vi "rx_top.vi"(0 "Received IQ\nwaveform":cluster{"t0":dbl, "dt":dbl, "Y":cdb[]} {"Y" format="%.2g"; "dt" format="%.2g"; "t0" format="%.2g"}, 2 "Modulation Parameters":T4 {"RX Parameters"."RX Sample Rate" items=["4M"]}, 4 "# of Receive Iterations":u16=1, 6 "stop":bool, 7 "error in":errorcluster) -> (9 "Received IQ Graph":cluster{dbl[], dbl[]}(graph) caption="IQ Graph", 10 "Received Magnitude":dbl[](graph), 11 "Received Constellation Graph":T7(graph) caption="Constellation Graph", 12 "Received Phase":dbl[](graph), 13 "Received Eye Diagram":cluster{"t0":dbl, "dt":dbl, "Y":dbl[]}[](graph) caption="Eye Diagram", 14 "coerced carrier frequency (Hz)":dbl format="%#_6p", 15 "Received I":waveform(dbl)(graph), 16 "coerced bandwidth":dbl, 17 "Received Q":waveform(dbl)(graph), 18 "coerced gain (dB)":dbl format="%#_6f", 19 "Received Power Spectrum Density":dbl[](graph), 20 "Measured channel impairements":T2, 21 "symbol rate":dbl format="%#_6p", 22 "offset":i32, 23 "overhead offset":i32, 24 "bit-error rate":dbl, 25 "average \nbit-error rate":dbl, 26 "key bit sequence":u8[](array[numeric]), 27 "error out":errorcluster)   [LabVIEW 2012]
uses:
  EE 497/LABS/SDR/control_type_defs.llb/rx_hw params.ctl
  EE 497/LABS/SDR/control_type_defs.llb/Queues.ctl
  <vilib>/Analysis/baseanly.llb/Mean (DBL).vi
  gds_hw_config.lvlib
  <vilib>/addons/Modulation/niAMT.lvlib
  <vilib>/Analysis/NI_AALBase.lvlib
panel:
  in  "Queues":T1
  out "Packet Detected":bool
  in  "Configurations":T3(tab)
  in  "HW parameters":T5={"Device IP Address"="192.168.11.6", "Active Antenna"="RX1", "Carrier Frequency (Hz)"=915000000.0, "Gain (dB)"=10.0, "Trigger Level"=0.01, "Bandwidth (Hz)"=40000000.0, "Reference Position (%)"=10.0, "Capture Time (s)"=0.0004, "Simulate"=FALSE} {"Capture Time (s)" format="%.2p"; "Bandwidth (Hz)" format="%.2p"; "Trigger Level" format="%#.3p"; "Gain (dB)" format="%.2f"; "Carrier Frequency (Hz)" format="%.2p"}
  in  "RX Graphs":T6(tab)
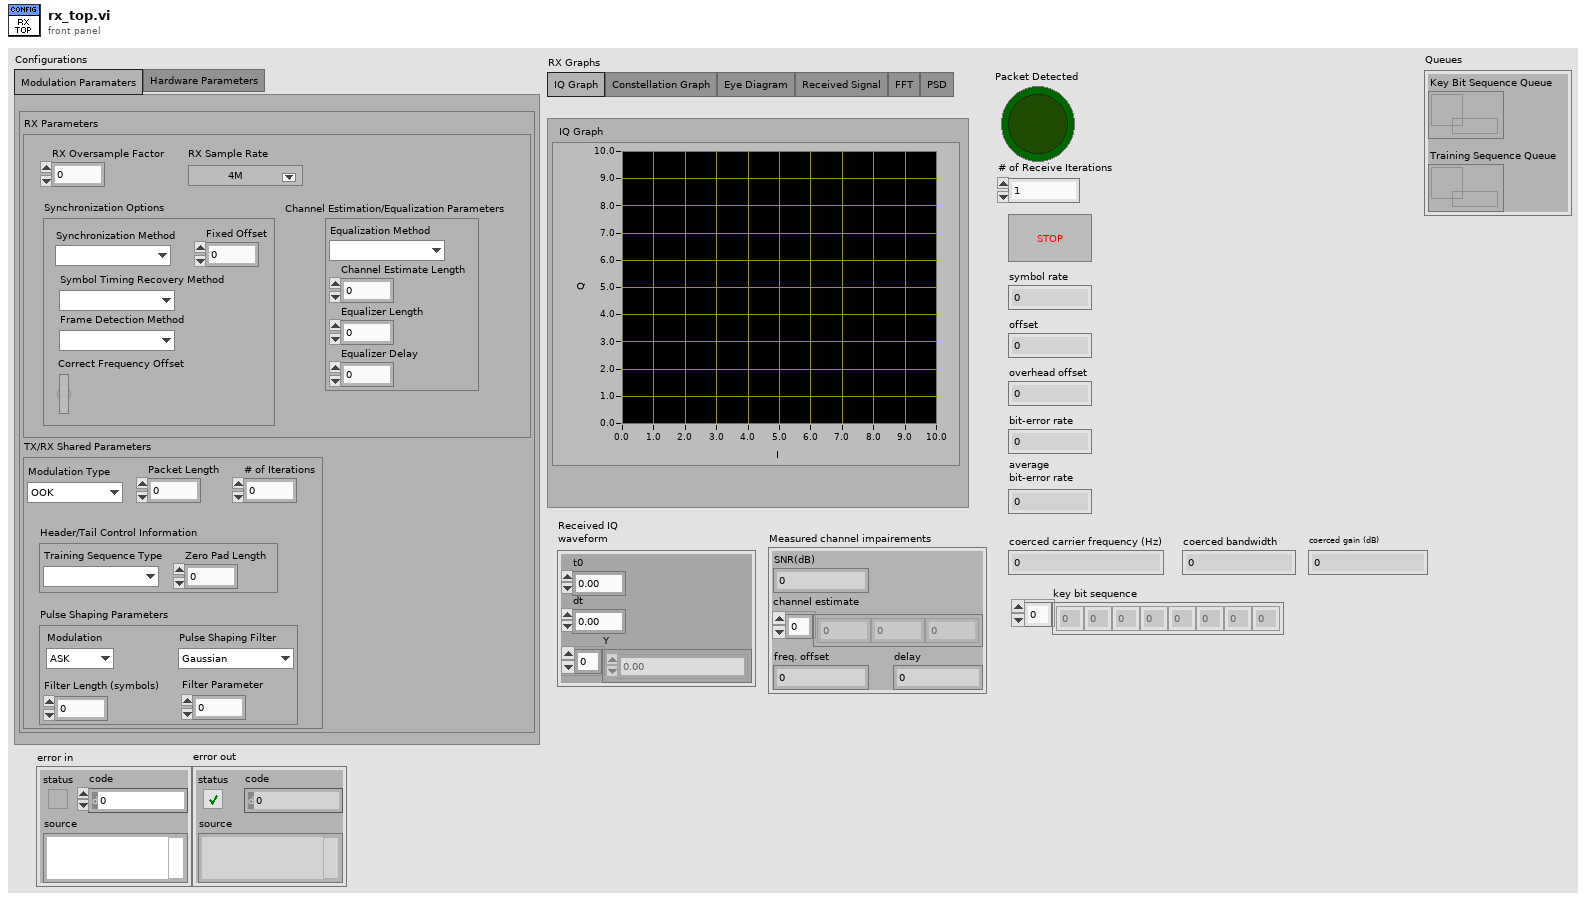
[diagram p1: front panel]
types:
  T1 = typedef "Queues.ctl" = cluster{"Key Bit Sequence Queue":refnum<queue>, "Training Sequence Queue":refnum<queue>}
  T2 = cluster{"SNR(dB)":dbl, "channel estimate":cdb[], "freq. offset":dbl, "delay":dbl}
  T3 = enum32{"Modulation Paramaters", "Hardware Parameters"}
  T4 = cluster{"RX Parameters":cluster{"RX Oversample Factor":dbl, "RX Sample Rate":dbl, "Synchronization Options":cluster{"Synchronization Method":enum16{""}, "Symbol Timing Recovery Method ":enum16{""}, "Fixed Offset":dbl, "Frame Detection Method":enum16{""}, "Correct Frequency Offset":bool}, "Channel Estimation/Equalization Parameters":cluster{"Equalization Method":enum16{""}, "Channel Estimate Length":dbl, "Equalizer Length":dbl, "Equalizer Delay":dbl}}, "TX/RX Shared Parameters":cluster{"Modulation Type":enum16{"OOK", "FSK"}, "Packet Length":dbl, "# of Iterations":dbl, "Pulse Shaping Parameters":cluster{"Modulation":enum16{"ASK", "FSK", "PSK", "QAM", "MSK", "PAM"}, "Pulse Shaping Filter":enum16{"Gaussian"}, "Filter Length (symbols)":dbl, "Filter Parameter":dbl}, "Header/Tail Control Information":cluster{"Training Sequence Type":enum16{""}, "Zero Pad Length":dbl}}}
  T5 = typedef "rx_hw params.ctl" = cluster{"Device IP Address":refnum<k15>, "Active Antenna":string, "Carrier Frequency (Hz)":dbl, "Gain (dB)":dbl, "Trigger Level":dbl, "Bandwidth (Hz)":dbl, "Reference Position (%)":dbl, "Capture Time (s)":dbl, "Simulate":bool}
  T6 = enum32{"IQ Graph", "Constellation Graph", "Eye Diagram", "Received Signal", "FFT", "PSD"}
  T7 = cluster{"Decimated Array":dbl[], "Decimated Array":dbl[]}[]
  T8 = cluster{"RX Oversample Factor":dbl, "RX Sample Rate":dbl, "Synchronization Options":cluster{"Synchronization Method":enum16{""}, "Symbol Timing Recovery Method ":enum16{""}, "Fixed Offset":dbl, "Frame Detection Method":enum16{""}, "Correct Frequency Offset":bool}, "Channel Estimation/Equalization Parameters":cluster{"Equalization Method":enum16{""}, "Channel Estimate Length":dbl, "Equalizer Length":dbl, "Equalizer Delay":dbl}}
  T9 = typedef "niAMT.lvlib/Complex Data Waveform.ctl" = cluster{"t0":dbl, "dt":dbl, "Y":cdb[]}
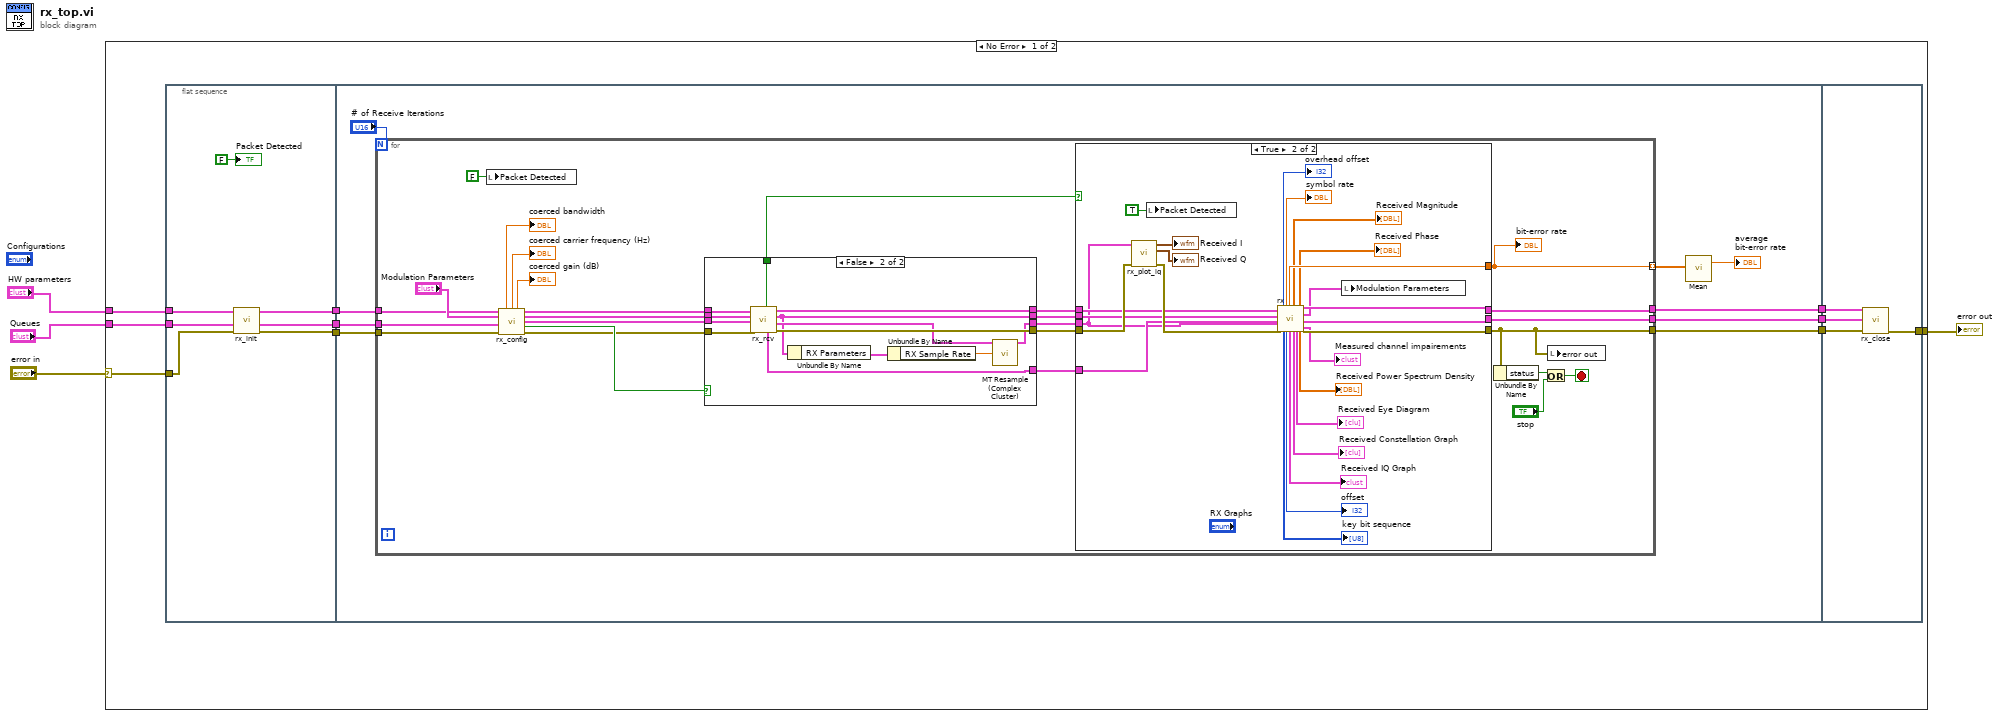
[diagram p0: block diagram]
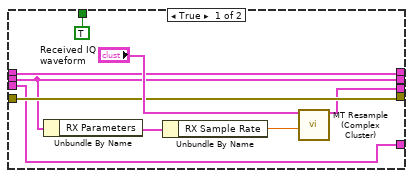
[diagram p3: hidden frame]
diagram:
  n1 = case shown="No Error" "error in" {
    selector: "error in" -> [w12 w111]
    tunnel: "HW parameters" -> [w14 _]
    tunnel: "Queues" -> [w13 _]
    tunnel: [w5 w111] -> w1
    frame No Error {
      n2 = flat-sequence {
        tunnel: w14 -> [w20]
        tunnel: w13 -> [w19]
        tunnel: w12 -> [w18]
        tunnel: [w17] -> w11
        tunnel: [w16] -> w10
        tunnel: [w15] -> w9
        tunnel: w11 -> [w29]
        tunnel: w10 -> [w28]
        tunnel: w9 -> [w27]
        tunnel: [w26] -> w8
        tunnel: [w25] -> w7
        tunnel: [w24] -> w6
        tunnel: w8 -> [w110]
        tunnel: w7 -> [w109]
        tunnel: w6 -> [w108]
        tunnel: [w107] -> w5
        frame #0 {
          n3 = call "rx_init.vi"("error in (no error)"=w18, "Queues in"=w19, "HW parameters In"=w20) -> ("error out"=w15:errorcluster, "Queues out"=w16:T1, "HW parameters Out"=w17:T5)  [unwired: 5 in, 1 out]
          "Packet Detected" <- FALSE ("Packet Detected")
        }
        frame #1 {
          n4 = for {
            N: "# of Receive Iterations" -> [_]
            tunnel: w29 -> [w54]
            tunnel: w28 -> [w53]
            tunnel: w27 -> [w52]
            tunnel: [w37] -> w26
            tunnel: [w32] -> w24
            tunnel: [w36] -> w25
            tunnel: [w31] -> w23 mode=indexing
            stop <- w33 stop-if-true
            n5 = local write "Packet Detected"(FALSE ("Packet Detected")) -> ()
            n6 = call "rx_config.vi"("HW parameters In"=w54, "Modulation Parameters In"="Modulation Parameters", "Queues In"=w53, "error in (no error)"=w52) -> ("coerced bandwidth"=→"coerced bandwidth":dbl, "coerced carrier frequency (Hz)"=→"coerced carrier frequency (Hz)":dbl, "coerced gain (dB)"=→"coerced gain (dB)":dbl, "HW parameters Out"=w47:T5, "Modulation Parameters Out"=w46:T4, "Queues Out"=w45:T1, "Simulate"=w48:bool, "error out"=w44:errorcluster)  [unwired: 4 in]
            n7 = case shown="False" w48 {
              tunnel: w47 -> [w91 w106]
              tunnel: w46 -> [w85 w105]
              tunnel: w45 -> [w89 w104]
              tunnel: w44 -> [w90 w103]
              tunnel: [w90 w100] -> w39
              tunnel: [w88 w94] -> w40
              tunnel: [w91 w98] -> w42
              tunnel: [w85 w97] -> w41
              tunnel: [TRUE ("Packet Detected") w96] -> w43
              tunnel: [w89 w95] -> w38
              frame True {
                n8 = Unbundle By Name(w85) -> ("RX Parameters"=w87:T8)
                n9 = Unbundle By Name(w87) -> ("RX Sample Rate"=w86:dbl)
                n10 = call <vilib>:"MT Resample (Complex Cluster).vi"("input complex waveform"="Received IQ\nwaveform", "desired sample rate (Hz)"=w86) -> ("output complex waveform"=w88:T9)  [unwired: 12 in, 1 out]
              }
              frame False {
                n11 = call "rx_rcv.vi"("error in (no error)"=w103, "Queues In"=w104, "Modulation Parameters In"=w105, "HW parameters In"=w106) -> ("error out"=w100:errorcluster, "Received IQ waveform"=w99:cluster{"t0":dbl, "dt":dbl, "Y":cdb[]}, "Modulation Parameters Out"=w97:T4, "HW parameters Out"=w98:T5, "Queues Out"=w95:T1, "Packet Detected"=w96:bool)  [unwired: 2 in]
                n12 = Unbundle By Name(w97) -> ("RX Parameters"=w102:T8)
                n13 = Unbundle By Name(w102) -> ("RX Sample Rate"=w101:dbl)
                n14 = call <vilib>:"MT Resample (Complex Cluster).vi"("input complex waveform"=w99, "desired sample rate (Hz)"=w101) -> ("output complex waveform"=w94:T9)  [unwired: 12 in, 1 out]
              }
            }
            n15 = case shown="True" w43 {
              tunnel: w42 -> [w59 w78]
              tunnel: w41 -> [_ w76]
              tunnel: w40 -> [_ w74]
              tunnel: w39 -> [w57 w80]
              tunnel: w38 -> [w58 w75]
              tunnel: [w59 w77] -> w37
              tunnel: [w58 w72] -> w36
              tunnel: [w57 w81] -> w32
              tunnel: [_ w73] -> w31
              frame False {
              }
              frame True {
                n16 = call "rx_plot_iq.vi"("error in"=w80, "Received IQ\nwaveform"=w74) -> ("error out"=w79:errorcluster, "Q component"=→"Received Q":waveform(dbl), "I component"=→"Received I":waveform(dbl))  [unwired: 7 in]
                n17 = local write "Packet Detected"(TRUE ("Packet Detected")) -> ()
                n18 = call "rx.vi"("HW parameters In"=w78, "Modulation Parameters In"=w76, "Queues In"=w75, "Received IQ\nwaveform"=w74, "error in (no error)"=w79) -> ("overhead offset"=→"overhead offset":i32, "key bit sequence"=→"key bit sequence":u8[], "symbol rate"=→"symbol rate":dbl, "offset"=→"offset":i32, "bit-error rate"=w73:dbl, "Received IQ Graph"=→"Received IQ Graph":cluster{dbl[], dbl[]}, "Received Magnitude"=→"Received Magnitude":dbl[], "Received Constellation Graph"=→"Received Constellation Graph":T7, "Received Eye Diagram"=→"Received Eye Diagram":cluster{"t0":dbl, "dt":dbl, "Y":dbl[]}[], "Received Phase"=→"Received Phase":dbl[], "Received Power Spectrum Density"=→"Received Power Spectrum Density":dbl[], "HW parameters Out"=w77:T5, "Modulation Parameters Out"=w71:T4, "Queues  Out"=w72:T1, "Measured channel impairements"=→"Measured channel impairements":T2, "error out"=w81:errorcluster)  [unwired: 7 in]
                n19 = local write "Modulation Parameters"(w71) -> ()
              }
            }
            "bit-error rate" <- w31
            n20 = Unbundle By Name(w32) -> ("status"=w35:bool)
            n21 = Or(x=w35, y="stop") -> (x .or. y?=w33:bool)
            n22 = local write "error out"(w32) -> ()
          }
          n23 = call-poly <vilib>:"Mean.vi"("X"=w23) -> ("mean"=→"average \nbit-error rate":dbl)  [unwired: 1 out]
        }
        frame #2 {
          n24 = call "rx_close.vi"("error in"=w108, "Queues"=w109, "HW parameters"=w110) -> ("error out"=w107:errorcluster)  [unwired: 8 in]
        }
      }
    }
    frame Error {
    }
  }
  "error out" <- w1
